vi "Shutdown.vi"(11 "API in":refnum<class "API.lvclass">) -> ()   [LabVIEW 2024, in "API.lvclass"]
uses:
  API.lvclass
  API.lvclass/API.ctl
  Message.ctl
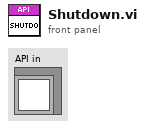
[diagram p1: front panel]
types:
  T1 = typedef "API.lvclass/Message.ctl" = cluster{"Name":string, "Data":variant}
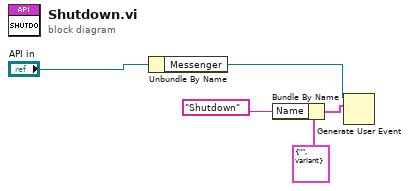
[diagram p0: block diagram]
diagram:
  n1 = Unbundle By Name("API in") -> ("Messenger"=w2:refnum<user-event>)
  n2 = Bundle By Name(cluster=T1 {"Name"="", "Data"=variant} ("Message"), "Name"="Shutdown") -> (w5:T1)
  n3 = Generate User Event(user event=w2, event data cluster=w5) -> ()  [unwired: 2 in, 2 out]
